vi "LSX Set Auto Limit After Calib RM.vi"(8 "error in (no error)":errorcluster, 10 "lFlags":i32, 11 "lLSID":i32) -> (0 "error out":errorcluster, 3 "function return":i32)   [LabVIEW 2018, in "Tango.lvlib"]
doc: "TANGOAPI int TANGOCALL LSX_SetAutoLimitAfterCalibRM (int lLSID, int lFlags);"
uses:
  Tango.lvlib
  SubVIs/Tango_DLL.dll
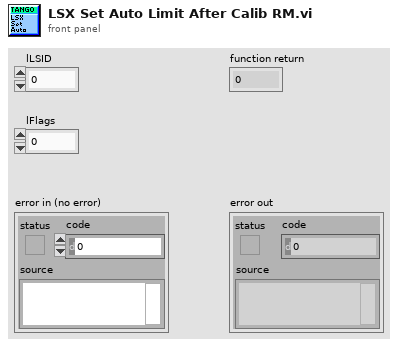
[diagram p1: front panel]
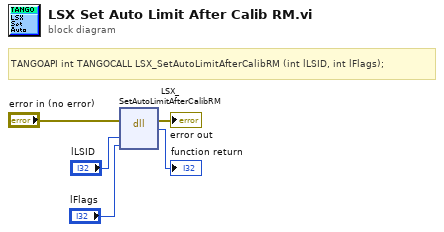
[diagram p0: block diagram]
diagram:
  # "TANGOAPI int TANGOCALL LSX_SetAutoLimitAfterCalibRM (int lLSID, int lFlags);"
  n1 = dll-call lib="C:/Users/Familie/Documents/LabviewIX81/lib/TANGO Stage/SubVIs/Tango_DLL.*" fn="LSX_SetAutoLimitAfterCalibRM"(error in="error in (no error)", "lLSID"="lLSID", "lFlags"="lFlags") -> (error out=→"error out":errorcluster, →"function return":i32)  [unwired: 4 in, 1 out]
